vi "onDestroy.vi"(8 "error in (no error)":errorcluster, 11 "DAQmx":refnum<class "DAQmx.lvclass">) -> (0 "error out":errorcluster, 3 "DAQmx out":refnum<class "DAQmx.lvclass">)   [LabVIEW 2019, in "DAQmx.lvclass"]
uses:
  DAQmx.lvclass
  <vilib>/JKI/JKI SMO/SMO/SMO.lvclass
panel:
  # "For instructions on how to use the JKI State Machine Objects, examples and video tutorials, visit:\nhttp://jki.net/state-machine-objects/\n\nJKI State Machine Objects™\nhttp://jki.net/state-machine-objects/\nCopyright (C) 2005-2015, JKI <info@jki.net>\nALL RIGHTS RESERVED"
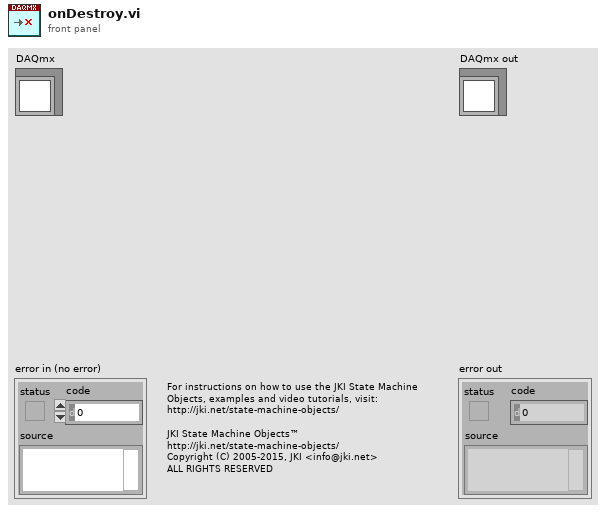
[diagram p1: front panel]
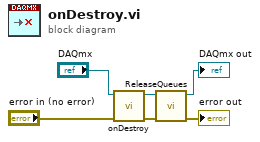
[diagram p0: block diagram]
diagram:
  n1 = call-parent "onDestroy.vi"("error in (no error)"="error in (no error)", "SMO"="DAQmx") -> ("error out"=w1:errorcluster, "SMO out"=w2:refnum<class "DAQmx.lvclass">)  [unwired: 8 in]
  n2 = call "ReleaseQueues.vi"("error in (no error)"=w1, "DAQmx"=w2) -> ("error out"=→"error out":errorcluster, "DAQmx out"=→"DAQmx out":refnum<class "DAQmx.lvclass">)  [unwired: 8 in]
